vi "EventFGV.vi"(5 "Action":enum16{"Set", "Get"}(ring)=enum."Get", 10 "user event in":refnum<user-event>) -> (2 "user event out":refnum<user-event>)   [LabVIEW 2017]
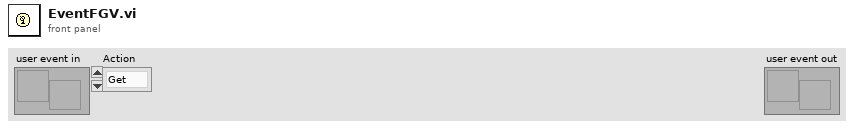
[diagram p1: front panel]
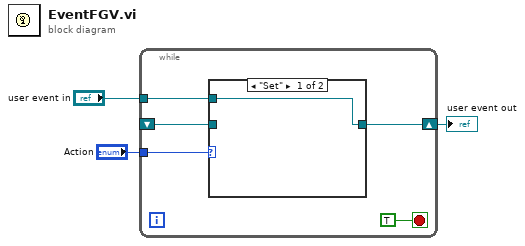
[diagram p0: block diagram]
diagram:
  n1 = while {
    shift-right: [w6] -> w1
    shift-left: _ -> [w5]
    tunnel: "Action" -> [w7]
    tunnel: "user event in" -> [w4]
    stop <- TRUE stop-if-true
    n2 = case shown="\"Set\"" w7 {
      tunnel: [w9 w10] -> w6
      tunnel: w5 -> [_ w10]
      tunnel: w4 -> [w9 _]
      frame "Set" {
      }
      frame "Get" {
      }
    }
  }
  "user event out" <- w1
